vi "Function and Derivative (VI).vi"(5 "sign":i32(ring) items=["y=f(x)", "y=-f(x)"], 6 "data":variant, 7 "f(x)":T1, 10 "(x+h)-x":dbl=1e-08 format="%.2e", 11 "x":dbl=1e-08 format="%.2e") -> (0 "error":i32, 2 "df(x)/dx":dbl format="%.2f", 3 "f(x)":dbl format="%.2f")   [LabVIEW 2014, in "NI_Gmath.lvlib"]
uses:
  NI_Gmath.lvlib
  functionRefnum.ctl
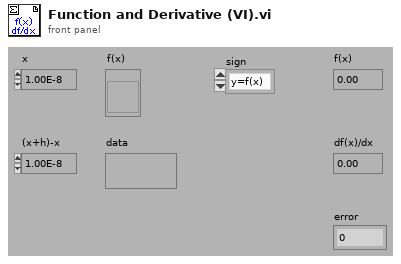
[diagram p1: front panel]
types:
  T1 = typedef "NI_Gmath.lvlib/functionRefnum.ctl" = refnum<vi>
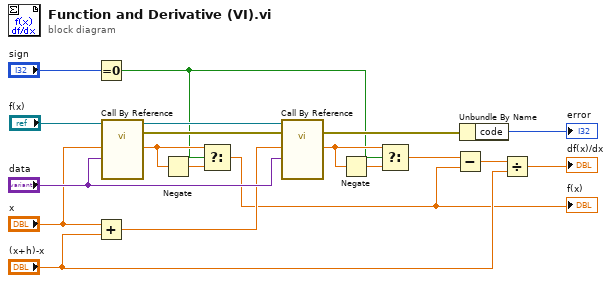
[diagram p0: block diagram]
diagram:
  n1 = Equal To 0?(x="sign") -> (x = 0?=w4:bool)
  n2 = Add(x="x", y="(x+h)-x") -> (x+y=w13:dbl)
  n3 = call-by-ref "?"(reference="f(x)", "Variant"="data", "x"="x") -> (reference out=w12:T1, error out=w19:errorcluster, 2:"f(x)"=w8:dbl)  [unwired: 4 in]
  n4 = Negate(x=w8) -> (-x=w7:dbl)
  n5 = Select(t=w8, s=w4, f=w7) -> (s? t:f=w2:dbl)
  "f(x)" <- w2
  n6 = call-by-ref "?"(reference=w12, error in=w19, "Variant"="data", "x"=w13) -> (error out=w18:errorcluster, "f(x)"=w5:dbl)  [unwired: 3 in, 1 out]
  n7 = Negate(x=w5) -> (-x=w6:dbl)
  n8 = Select(t=w5, s=w4, f=w6) -> (s? t:f=w3:dbl)
  n9 = Subtract(x=w3, y=w2) -> (x-y=w1:dbl)
  n10 = Unbundle By Name(w18) -> ("code"=→"error":i32)
  n11 = Divide(x=w1, y="(x+h)-x") -> (x/y=→"df(x)/dx":dbl)
